vi "ex2_TotalDAQ.vi"() -> ()   [LabVIEW 2010]
panel:
  out "DeviceID":string
  out "DeviceConnection":bool
  out "Status Information":string
  in  "Acquire Start":bool
  out "CH2 Data":dbl[](graph)
  out "CH1 Data":dbl[](graph)
  in  "Acquire Stop":bool
  in  "Exit":bool
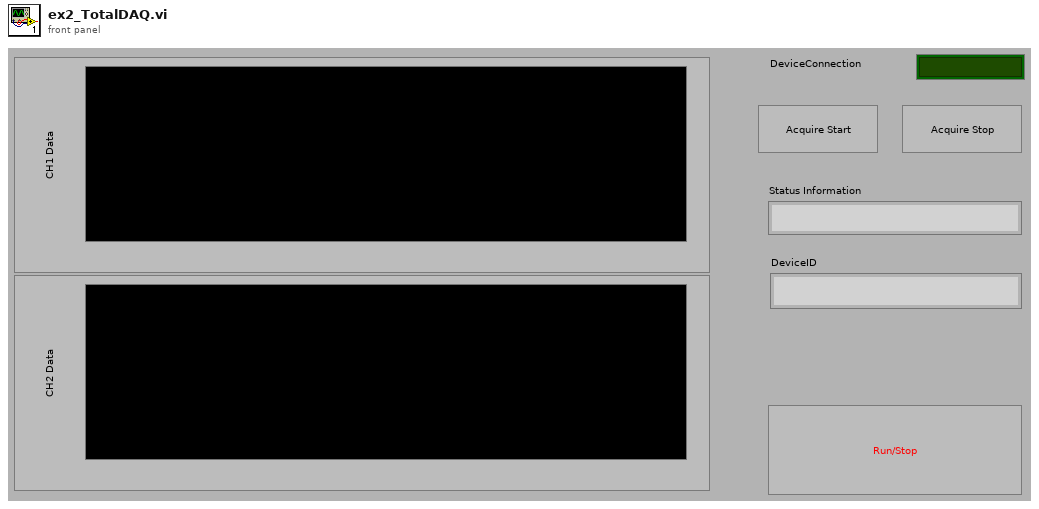
[diagram p1: front panel]
types:
  T1 = cluster{"Q_DblData":refnum<queue>, "DeviceHandle":u32, "Q_EventData":refnum<queue>, "Q_Int16Data":refnum<queue>}
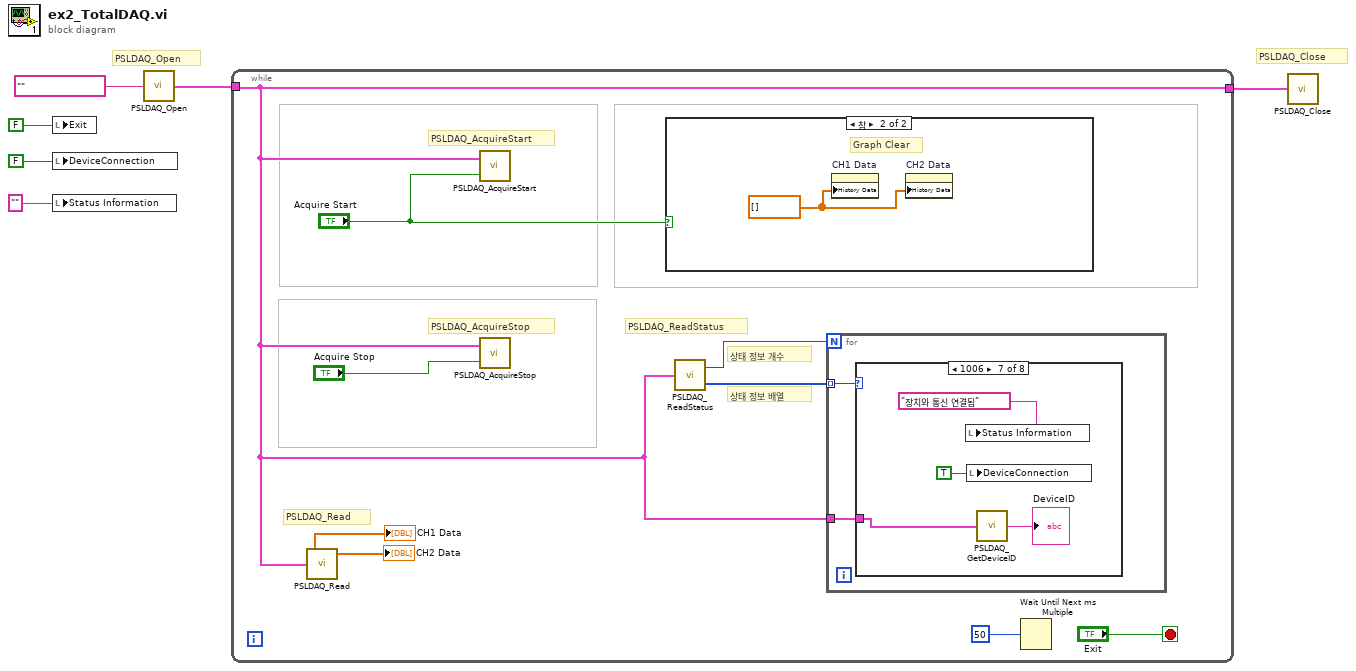
[diagram p0: block diagram]
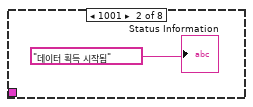
[diagram p3: hidden frame]
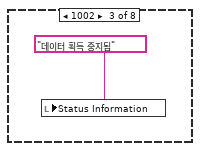
[diagram p4: hidden frame]
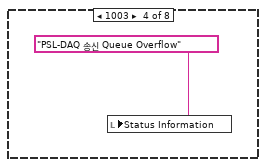
[diagram p5: hidden frame]
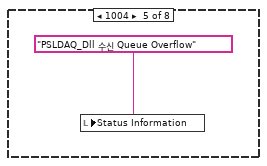
[diagram p6: hidden frame]
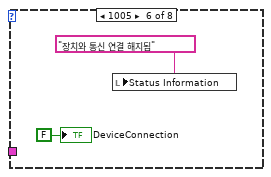
[diagram p7: hidden frame]
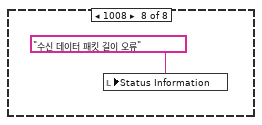
[diagram p8: hidden frame]
diagram:
  # "PSLDAQ_Close"
  # "PSLDAQ_Open"
  n1 = local write "Exit"(FALSE ("Run Stop")) -> ()
  n2 = local write "DeviceConnection"(FALSE ("DeviceConnect")) -> ()
  n3 = local write "Status Information"("" ("Status Information")) -> ()
  n4 = call "PSLDAQ_Open.vi"("DeviceID"="" ("DeviceName")) -> ("Handle Out"=w2:T1)
  n5 = while {
    tunnel: [w7] -> w1
    tunnel: w2 -> [w7]
    stop <- "Exit" stop-if-true
    # "PSLDAQ_Read"
    # "PSLDAQ_AcquireStop"
    # "상태 정보 개수"
    # "PSLDAQ_ReadStatus"
    # "상태 정보 배열"
    # "PSLDAQ_AcquireStart"
    n6 = call "PSLDAQ_Read.vi"("Handle In"=w7) -> ("CH2 Data"=→"CH2 Data":dbl[], "CH1 Data"=→"CH1 Data":dbl[])  [unwired: 3 out]
    n7 = call "PSLDAQ_AcquireStart.vi"("Trigger"="Acquire Start", "Handle In"=w7) -> ()  [unwired: 1 in]
    n8 = call "PSLDAQ_AcquireStop.vi"("Trigger"="Acquire Stop", "Handle In"=w7) -> ()  [unwired: 1 in]
    n9 = case shown="참" "Acquire Start" {
      frame False {
      }
      frame True {
        w29 = dbl[] [] ("History Data")
        # "Graph Clear"
        n10 = property on="CH1 Data" class="WFChart (엄격한)"("History Data"=w29) -> ()  [unwired: 2 in, 2 out]
        n11 = property on="CH2 Data" class="WFChart (엄격한)"("History Data"=w29) -> ()  [unwired: 2 in, 2 out]
      }
    }
    n12 = call "PSLDAQ_ReadStatus.vi"("Handle In"=w7) -> ("Status"=w11:u32[], "# Read"=w10:i32)
    n13 = for {
      N: w10 -> [_]
      tunnel: w7 -> [w17]
      tunnel: w11 -> [w16] mode=indexing
      n14 = case shown="1006" w16 {
        tunnel: w17 -> [_ _ _ _ _ _ w25 _]
        frame 0, Default {
        }
        frame 1001 {
          "Status Information" <- "데이터 획득 시작됨" ("Status Information")
        }
        frame 1002 {
          n15 = local write "Status Information"("데이터 획득 중지됨" ("Status Information")) -> ()
        }
        frame 1003 {
          n16 = local write "Status Information"("PSL-DAQ 송신 Queue Overflow" ("Status Information")) -> ()
        }
        frame 1004 {
          n17 = local write "Status Information"("PSLDAQ_Dll 수신 Queue Overflow" ("Status Information")) -> ()
        }
        frame 1005 {
          n18 = local write "Status Information"("장치와 통신 연결 해지됨" ("Status Information")) -> ()
          "DeviceConnection" <- FALSE ("DeviceConnect")
        }
        frame 1006 {
          n19 = local write "Status Information"("장치와 통신 연결됨" ("Status Information")) -> ()
          n20 = local write "DeviceConnection"(TRUE ("DeviceConnect")) -> ()
          n21 = call "PSLDAQ_GetDeviceID.vi"("Handle In"=w25) -> ("DeviceID"=→"DeviceID":string)
        }
        frame 1008 {
          n22 = local write "Status Information"("수신 데이터 패킷 길이 오류" ("Status Information")) -> ()
        }
      }
    }
    n23 = Wait Until Next ms Multiple(millisecond multiple=u32 50) -> ()  [unwired: 1 out]
  }
  n24 = call "PSLDAQ_Close.vi"("Handle In"=w1) -> ()
